vi "Compute Z from Disparity.vi"(2 "Xr":dbl, 3 "Xl":dbl, 4 "f":dbl=4.4, 5 "b":dbl=254.0) -> (0 "Zft":dbl, 1 "Z":dbl)   [LabVIEW 2011]
panel:
  out "d":dbl
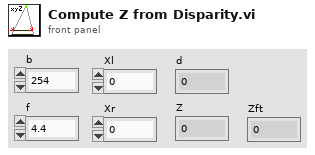
[diagram p1: front panel]
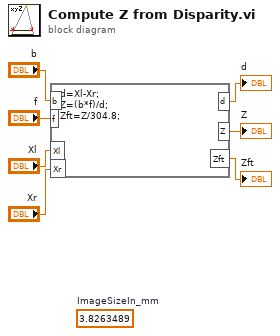
[diagram p0: block diagram]
diagram:
  (unwired) 3.8263489  # ImageSizeIn_mm
  n1 = formula code="d=Xl-Xr;\nZ=(b*f)/d;\nZft=Z/304.8;"("b"="b", "f"="f", "Xl"="Xl", "Xr"="Xr") -> ("Z"=→"Z":dbl, "d"=→"d":dbl, "Zft"=→"Zft":dbl)
